vi "For force-activate and assembly exp.vi"() -> ()   [LabVIEW 2014]
panel:
  in  "Set Force (pN)":dbl=46.5 format="%_8g"
  in  "Avg points":i32=120
  in  "feedback moving step size (um)":dbl=0.03
  in  "pFC FEC range (um)":dbl=3.1500000000000012 format="%.3f"
  in  "pFC feedback?":bool=TRUE
  in  "save pFC?":bool=TRUE
  in  "Set LaserPower for activate (mV)":dbl=-3500.0 format="%0.2f"
  in  "Who's Data":enum16{"YCC", "PYW", "LCH", "YYH"}(ring)
  in  "File name add to the end \n(laser power-height)":string="FA-h300-1 uM m51 BRC4-Ca-K250-2-2"
  in  "Record scan rate  (um/s)":dbl=2.0 format="%.3f"
  in  "range  (um)":dbl=3.000000000000002 format="%.3f"
  in  "T=X\nF=Y":bool=TRUE
  # "0.33V for h300 and 1200mV power"
  # "FA-h300-1 uM m51 BRC4-Ca-K250-2-2"
  # "FA-h300-1 uM m51-KCl 250-Ca-1-7"
  # "FA-h300-1 uM m51 and S5S1-Ca-ATP-1-4"
  # "FA-h300-1 uM m51-Ca-2-1"
  # "FA-h300-1 uM m51-Mg-AMPPNP-2-3"
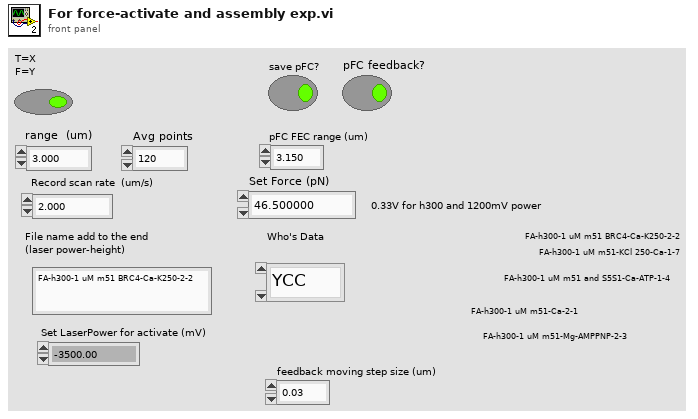
[diagram p1: front panel]
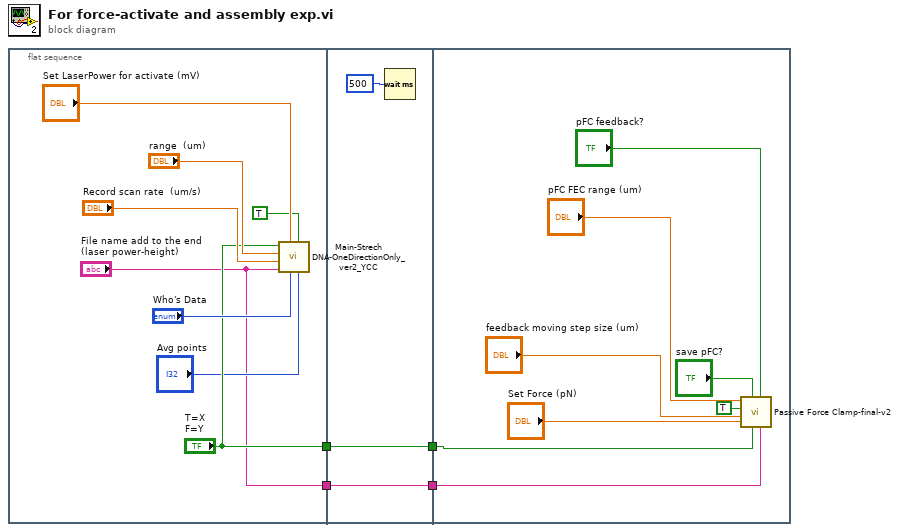
[diagram p0: block diagram]
diagram:
  n1 = flat-sequence {
    tunnel: ["T=X\nF=Y"] -> w4
    tunnel: ["File name add to the end \n(laser power-height)"] -> w1
    tunnel: w4 -> [w15]
    tunnel: [w15] -> w3
    tunnel: [w13] -> w2
    tunnel: w1 -> [w13]
    tunnel: w3 -> [w20]
    tunnel: w2 -> [w16]
    frame #0 {
      n2 = call "Main-Strech DNA-OneDirectionOnly_ver2_YCC.vi"("Avg points"="Avg points", "Save Data?"=TRUE, "Who's Data"="Who's Data", "Set LaserPower (mV)"="Set LaserPower for activate (mV)", "File name add to the end \n(laser power-height)"="File name add to the end \n(laser power-height)", "Record scan rate  (um/s)"="Record scan rate  (um/s)", "range  (um)"="range  (um)", "T=X\nF=Y"="T=X\nF=Y") -> ()  [unwired: 3 in, 1 out]
    }
    frame #1 {
      n3 = Wait (ms)(milliseconds to wait=u32 500) -> ()  [unwired: 1 out]
    }
    frame #2 {
      n4 = call "Passive Force Clamp-final-v2.vi"("file name add to the end (height)"=w16, "feedback?"="pFC feedback?", "X=T,Y=F"=w20, "save?"="save pFC?", "Set Force (pN)"="Set Force (pN)", "moving step size (um)"="feedback moving step size (um)", "Auto Find"=TRUE, "range (um)"="pFC FEC range (um)") -> ()  [unwired: 4 in]
    }
  }
